vi "ConsoleHeader.vi"() -> (0 "Console Header":string)   [LabVIEW 2012]
uses:
  <userlib>/ROSforLV/ROS/Code/_ROSDefinition.vi
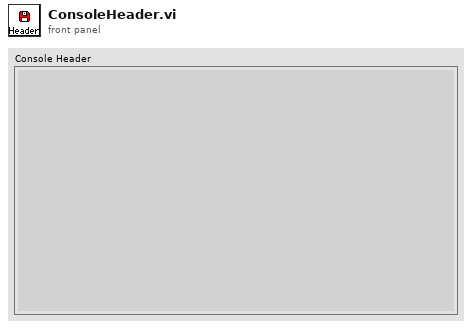
[diagram p1: front panel]
types:
  T1 = enum16{"Add Server", "Clear Server", "Clear All", "Get Info", "GetPanelInfo"}
  T2 = enum16{"http://IP:port", "http://IP", "IP:port", "IP only"}
  T3 = typedef "MyState.ctl" = enum16{"No Connection", "Registered", "Connected", "Close"}
  T4 = typedef "ServoInfo.ctl" = cluster{"vi name":string, "VI Refnum":refnum<vi>, "queue":refnum<queue>, "ROS":T5, "notifier":refnum<notifier>}
  T5 = typedef "_ROSControl.ctl" = cluster{"topic port":u16, "Node":string, "topic":string, "type":string, "node port":u16, "error ":errorcluster, "Direction":T6, "APIs":string[], "Update (ms)":u16, "write queue":u16}
  T6 = typedef "_ROSDirection.ctl" = enum16{"Node", "Publisher", "Subscriber", "Service Client"}
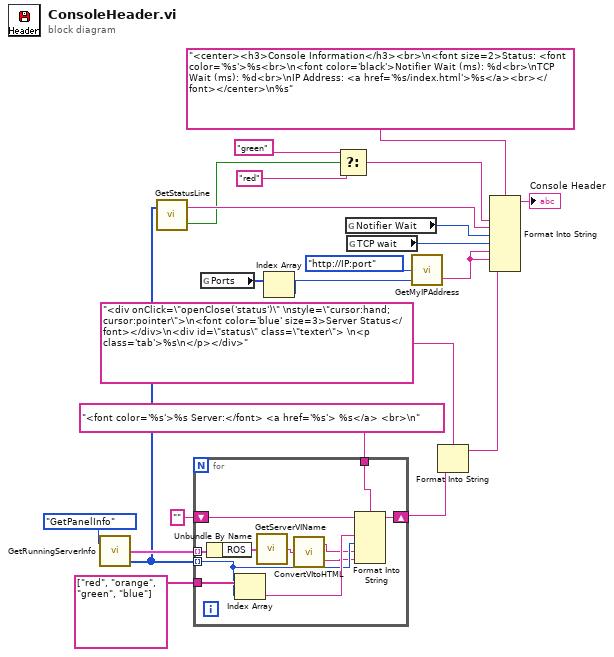
[diagram p0: block diagram]
diagram:
  n1 = call <userlib>:"GetRunningServerInfo.vi"("Task"=T1."GetPanelInfo") -> ("Status"=w7:T3[], "servers"=w13:T4[])  [unwired: 1 in, 1 out]
  n2 = call <userlib>:"GetStatusLine.vi"("Status"=w7) -> ("all good?"=w6:bool, "Status"=w8:string)  [unwired: 1 in]
  n3 = for {
    tunnel: w13 -> [w33] mode=indexing
    tunnel: w7 -> [w25] mode=indexing
    shift-right: [w31] -> w11
    shift-left: "" -> [w32]
    tunnel: "<font color='%s'>%s Server:</font> <a href='%s'> %s</a> <br>\n" -> [w30]
    tunnel: string[] ["red", "orange", "green", "blue"] -> [w29]
    n4 = Unbundle By Name(w33) -> ("ROS"=w28:T5)
    n5 = Index Array(array=w29, index=w25) -> (element=w26:string)
    n6 = call <userlib>:"GetServerVIName.vi"("ROS"=w28) -> ("vi name"=w27:string)
    n7 = call <userlib>:"ConvertVItoHTML.vi"("vi name"=w27) -> ("Htm log name"=w24:string, "Server Name"=w23:string)
    n8 = Format Into String(format string=w30, initial string=w32, w26, w25, w24, w23) -> (resulting string=w31:string)  [unwired: 1 in, 1 out]
  }
  n9 = global read "_ROSDefinition.vi" "Ports"() -> (w4:u16[])
  n10 = Index Array(array=w4) -> (element=w3:u16)  [unwired: 1 in]
  n11 = Select(t="green", s=w6, f="red") -> (s? t:f=w16:string)
  n12 = global read "_ROSDefinition.vi" "Notifier Wait"() -> (w20:i32)
  n13 = global read "_ROSDefinition.vi" "TCP wait"() -> (w21:i32)
  n14 = call <userlib>:"GetMyIPAddress.vi"("Port"=w3, "Format"=T2."http://IP:port") -> ("URI"=w1:string)  [unwired: 2 in]
  n15 = Format Into String(format string="<div onClick=\"openClose('status')\" \nstyle=\"cursor:hand; cursor:pointer\">\n<font color='blue' size=3>Server Status</font></div>\n<div id=\"status\" class=\"texter\"> \n<p class='tab'>%s\n</p></div>" ("string"), w11) -> (resulting string=w2:string)  [unwired: 2 in, 1 out]
  n16 = Format Into String(format string="<center><h3>Console Information</h3><br>\n<font size=2>Status: <font color='%s'>%s<br>\n<font color='black'>Notifier Wait (ms): %d<br>\nTCP Wait (ms): %d<br>\nIP Address: <a href='%s/index.html'>%s</a><br></font></center>\n%s" ("Console Info"), w16, w8, w20, w21, w1, w1, w2) -> (resulting string=→"Console Header":string)  [unwired: 2 in, 1 out]
